vi "SP Figure Waveform Query Strings from Display Controls.vi"(4 "error in (no error)":errorcluster, 7 "CH Control":T1={"Trace On"=TRUE, "Measure"=0, "Format"=0, "Autoscale"=TRUE, "Reference"=0.0, "\nRefUnit"="dB/Div", "Position"=5.0, "Scale"=10.0, "ScaleUnit"="dB/Div", "LimitOn"=TRUE, "LimitFill"=FALSE, "Display Data"=0, "Show Markers"=TRUE, "SXX"=""} {"Measure" items=["S11", "S21", "S12", "S22"]; "Reference" format="%#.2g"; "Display Data" items=["Data", "Memory", "Data/Memory"]; "Format" items=["Log Mag", "Phase", "Expanded Phase", "Delay", "Smith", "Polar", "Lin Mag", "SWR", "Loss", "Real", "Imaginary"]; "Scale" min=0.001 step=1.0 format="%#.2g"; "Position" min=0.0 max=10.0}) -> (0 "error out":errorcluster, 1 "Limit Format":T4, 3 "Waveform Names":string[](array[string]))   [LabVIEW 2011]
uses:
  TypeDefs/SP Format.ctl
  TypeDefs/SP Display Trace Controls.ctl
  TypeDefs/SP Display Format.ctl
  TypeDefs/SP Display Data.ctl
panel:
  # "Div"
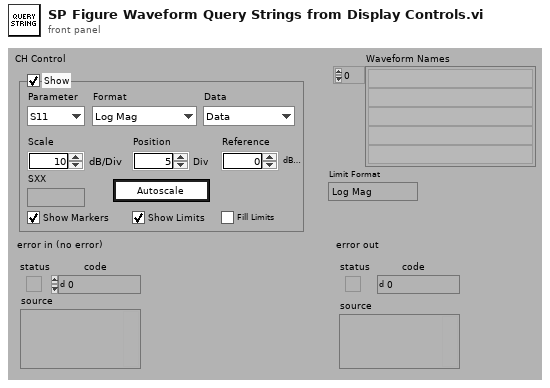
[diagram p1: front panel]
types:
  T1 = typedef "SP Display Trace Controls.ctl" = cluster{"Trace On":bool, "Measure":i32, "Format":T2, "Autoscale":bool, "Reference":dbl, "\nRefUnit":string, "Position":dbl, "Scale":dbl, "ScaleUnit":string, "LimitOn":bool, "LimitFill":bool, "Display Data":T3, "Show Markers":bool, "SXX":string}
  T2 = typedef "SP Display Format.ctl" = i32
  T3 = typedef "SP Display Data.ctl" = u16
  T4 = typedef "SP Format.ctl" = enum16{"Log Mag", "Lin Mag", "SWR", "Phase", "Expanded Phase", "Delay", "Insertion Loss", "Isolation", "Return Loss"}
  T5 = typedef "SP Parameter.ctl" = cluster{"Stimulus Port":i8, "Response Port":i8}
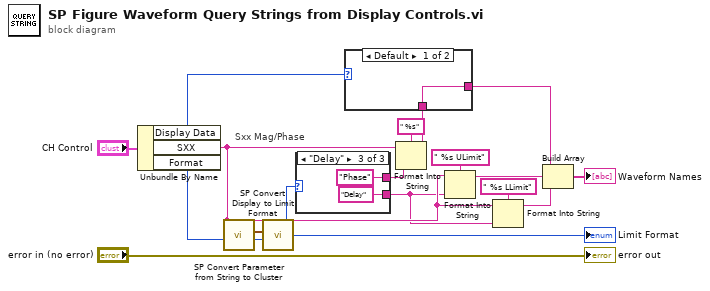
[diagram p0: block diagram]
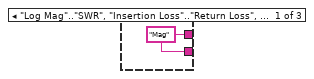
[diagram p2: hidden frame]
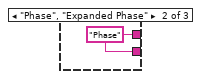
[diagram p3: hidden frame]
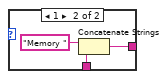
[diagram p4: hidden frame]
diagram:
  # "Sxx Mag/Phase"
  n1 = Unbundle By Name("CH Control") -> ("Display Data"=w15:T3, "SXX"=w5:string, "Format"=w12:T2)
  n2 = call "SP Convert Parameter from String to Cluster.vi"("Parameter String"=w5) -> ("Parameter"=w11:T5)  [unwired: 10 out]
  n3 = call "SP Convert Display to Limit Format.vi"("Display Format"=w12, "S Parameter"=w11) -> ("Limit Format"=w10:T4)  [unwired: 4 out]
  "Limit Format" <- w10
  n4 = case shown="\"Delay\"" w10 {
    tunnel: [w18 w19 "Phase"] -> w9
    tunnel: [w18 w19 "Delay"] -> w3
    frame "Log Mag".."SWR", "Insertion Loss".."Return Loss", Default {
      w18 = "Mag"
    }
    frame "Phase", "Expanded Phase" {
      w19 = "Phase"
    }
    frame "Delay" {
    }
  }
  n5 = Format Into String(format string=" %s", initial string=w5, w9) -> (resulting string=w8:string)  [unwired: 1 in, 1 out]
  n6 = case shown="Default" w15 {
    tunnel: w8 -> [w22 w25]
    tunnel: [w22 w23] -> w13
    frame Default {
    }
    frame 1 {
      n7 = Concatenate Strings("Memory " ("element"), w25) -> (w23:string)
    }
  }
  n8 = Format Into String(format string=" %s ULimit", initial string=w5, w3) -> (resulting string=w6:string)  [unwired: 1 in, 1 out]
  n9 = Format Into String(format string=" %s LLimit", initial string=w5, w3) -> (resulting string=w7:string)  [unwired: 1 in, 1 out]
  n10 = Build Array(w13, w6, w7) -> (→"Waveform Names":string[])
  "error out" <- "error in (no error)"
